vi "Run Main VI Core.vi"(8 "error in (no error)":errorcluster, 11 "Calling VI Ref in":refnum<vi>) -> (0 "error out":errorcluster, 3 "Calling VI Ref out":refnum<vi>)   [LabVIEW 2016]
uses:
  <vilib>/regexp/Match Regular Expression.xnode
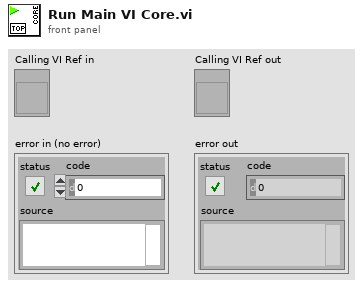
[diagram p1: front panel]
types:
  T1 = enum32{"Invalid", "Standard", "Closed", "Hidden", "Minimized", "Maximized"}
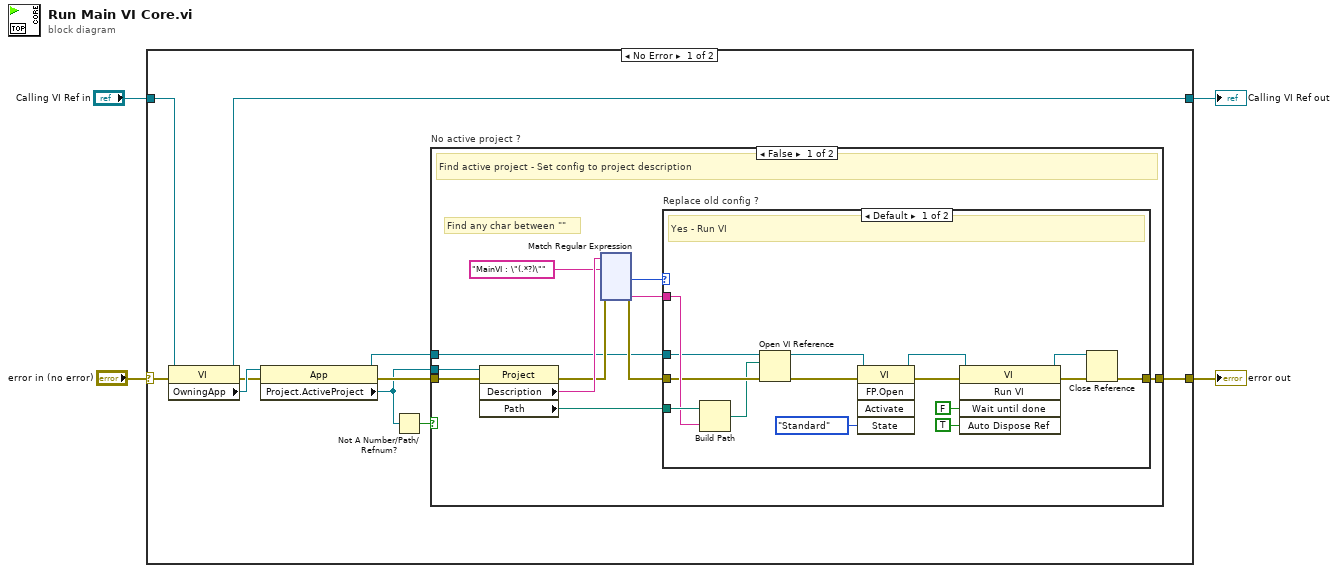
[diagram p0: block diagram]
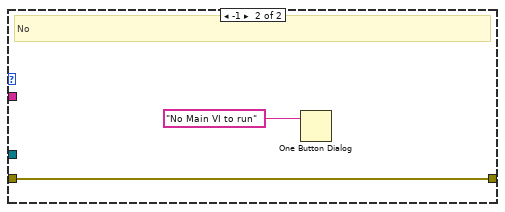
[diagram p2: hidden frame]
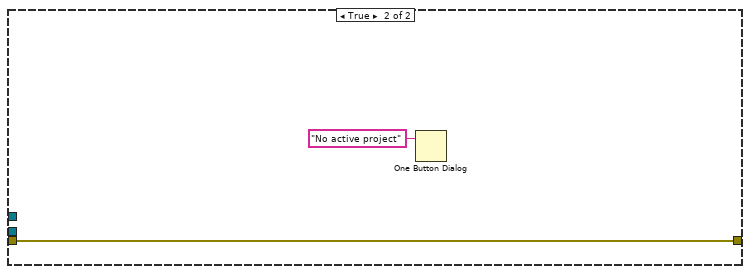
[diagram p3: hidden frame]
diagram:
  n1 = case shown="No Error" "error in (no error)" {
    selector: "error in (no error)" -> [w11 w162]
    tunnel: [w9 w162] -> w3
    tunnel: "Calling VI Ref in" -> [w10 w161]
    tunnel: [w8 w161] -> w1
    frame No Error {
      n2 = property class="VI"(reference=w10, error in=w11) -> (reference out=w8:refnum<vi>, error out=w13:errorcluster, "OwningApp"=w14:refnum<vi>)
      n3 = property class="App"(reference=w14, error in=w13) -> (reference out=w5:refnum<vi>, error out=w7:errorcluster, "Project.ActiveProject"=w6:refnum<vi>)
      n4 = Not A Number/Path/Refnum?(number/path/refnum=w6) -> (NaN/Path/Refnum?=w12:bool)
      n5 = case "No active project ?" shown="False" w12 {
        tunnel: w7 -> [w25 w159]
        tunnel: [w17 w159] -> w9
        tunnel: w6 -> [w24 _]
        tunnel: w5 -> [w15 _]
        frame False {
          # "Find any char between \"\""
          # "Find active project - Set config to project description"
          n6 = property class="Project"(reference=w24, error in=w25) -> (error out=w22:errorcluster, "Description"=w23:string, "Path"=w16:path)  [unwired: 1 out]
          n7 = xnode "Match Regular Expression"("input string"=w23, "regular expression"="MainVI : \"(.*?)\"", "error in"=w22) -> ("offset past match"=w18:i32, "error out"=w21:errorcluster, "submatch 1"=w19:string)  [unwired: 3 in, 3 out]
          n8 = case "Replace old config ?" shown="Default" w18 {
            tunnel: [w151 w157] -> w17
            tunnel: w21 -> [w154 w157]
            tunnel: w19 -> [w155 _]
            tunnel: w16 -> [w156 _]
            tunnel: w15 -> [w142 _]
            frame Default {
              # "Yes - Run VI"
              n9 = Build Path(base path=w156, name or relative path=w155) -> (appended path=w153:path)
              n10 = Open VI Reference(application reference (local)=w142, vi path=w153, error in (no error)=w154) -> (vi reference=w145:refnum<vi>, error out=w147:errorcluster)  [unwired: 3 in]
              n11 = invoke class="VI" method="FP.Open"(reference=w145, error in=w147, "State"=T1."Standard") -> (reference out=w144:refnum<vi>, error out=w146:errorcluster)  [unwired: 2 in, 3 out]
              n12 = invoke class="VI" method="Run VI"(reference=w144, error in=w146, "Wait until done"=FALSE ("Wait Until Done"), "Auto Dispose Ref"=TRUE ("Auto Dispose Reference")) -> (reference out=w150:refnum<vi>, error out=w152:errorcluster)  [unwired: 1 in, 3 out]
              n13 = Close Reference(reference=w150, error in (no error)=w152) -> (error out=w151:errorcluster)
            }
            frame -1 {
              # "No"
              n14 = One Button Dialog(message="No Main VI to run") -> ()  [unwired: 1 in, 1 out]
            }
          }
        }
        frame True {
          n15 = One Button Dialog(message="No active project") -> ()  [unwired: 1 in, 1 out]
        }
      }
    }
    frame Error {
    }
  }
  "error out" <- w3
  "Calling VI Ref out" <- w1
